vi "Motion-Intialize-Drives.vi"(8 "error in (no error)":errorcluster, 11 "Motion-ControlAll in":refnum<class "Motion-ControlAll.lvclass">) -> (0 "error out":errorcluster, 3 "Motion-ControlAll out":refnum<class "Motion-ControlAll.lvclass">)   [LabVIEW 2013, in "Motion-ControlAll.lvclass"]
uses:
  Motion-ControlAll.lvclass
  Motion-ControlAll.lvclass/Motion-ControlAll.ctl
  <vilib>/addons/_LabVIEW Style Book/Utilities/Style Book Utilities.lvlib
panel:
  out "Normalizing Data":u8(slide) scale=0.0..38.0
  out "STOP":bool
  # "Please wait while Motors Initialize"
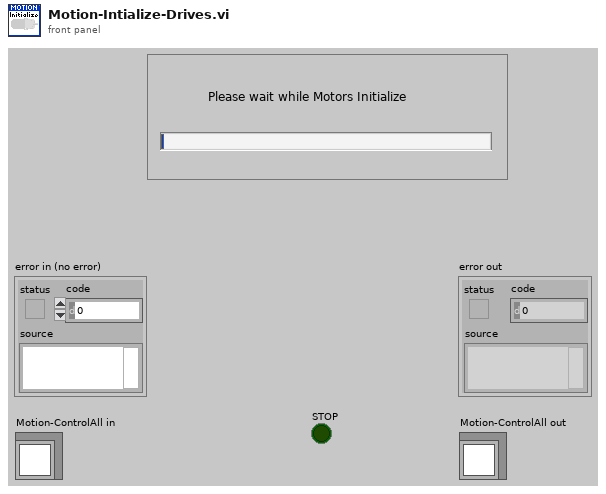
[diagram p1: front panel]
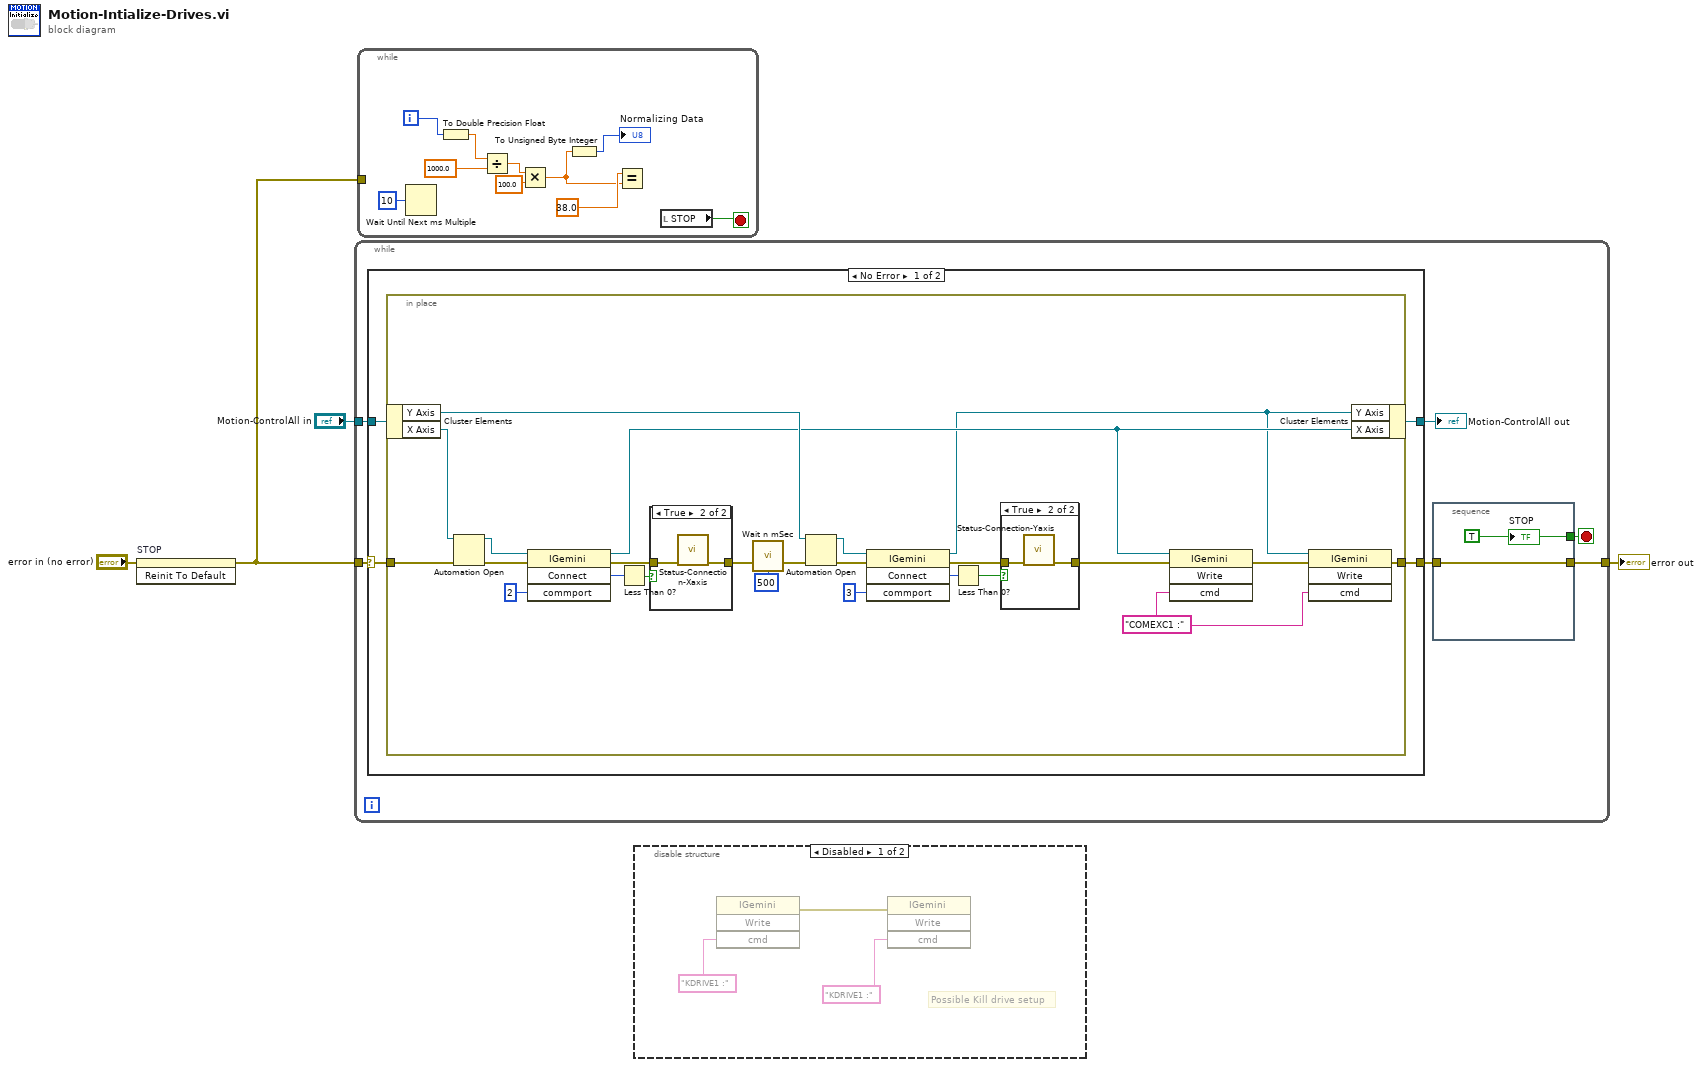
[diagram p0: block diagram]
diagram:
  n1 = invoke on="STOP" class="Bool (strict)" method="Reinit To Default"(error in="error in (no error)") -> (error out=w1:errorcluster)  [unwired: 2 in, 2 out]
  n2 = while {
    tunnel: w1 -> [w9]
    tunnel: [w6] -> w4
    tunnel: "Motion-ControlAll in" -> [w5]
    stop <- w7 stop-if-true
    n3 = case shown="No Error" w9 {
      selector: w9 -> [w15 w48]
      tunnel: [w14 w48] -> w8
      tunnel: [w13 w47] -> w10
      tunnel: w5 -> [w16 w47]
      frame No Error {
        n4 = in-place {
          in-place-border: w15 -> [w40]
          in-place-border: [w31] -> w14
          w33 = "COMEXC1 :" ("cmd")
          n5 = in-place-cluster #1(w16) -> ("Y Axis"=w22:refnum<k7>, "X Axis"=w32:refnum<k7>)
          n6 = Automation Open(error in (no error)=w40, Automation Refnum=w32) -> (Automation Refnum=w37:refnum<k7>, error out=w38:errorcluster)  [unwired: 2 in]
          n7 = invoke class="IGemini" method="Connect"(reference=w37, error in=w38, "commport"=i16 2) -> (reference out=w21:refnum<k7>, error out=w36:errorcluster, "Connect"=w35:i16)  [unwired: 1 in, 1 out]
          n8 = Less Than 0?(x=w35) -> (x < 0?=w30:bool)
          n9 = case shown="True" w30 {
            tunnel: w36 -> [w44 w46]
            tunnel: [w44 w45] -> w19
            frame False {
            }
            frame True {
              n10 = call "Status-Connection-Xaxis.vi"("error in"=w46) -> ("error out"=w45:errorcluster)  [unwired: 10 in]
            }
          }
          n11 = call <vilib>:"Wait n mSec.vi"("error in (no error)"=w19, "Milliseconds to Wait (500)"=u32 500) -> ("error out"=w18:errorcluster)  [unwired: 13 in]
          n12 = Automation Open(error in (no error)=w18, Automation Refnum=w22) -> (Automation Refnum=w26:refnum<k7>, error out=w27:errorcluster)  [unwired: 2 in]
          n13 = invoke class="IGemini" method="Connect"(reference=w26, error in=w27, "commport"=i16 3) -> (reference out=w20:refnum<k7>, error out=w24:errorcluster, "Connect"=w29:i16)  [unwired: 1 in, 1 out]
          n14 = Less Than 0?(x=w29) -> (x < 0?=w25:bool)
          n15 = case shown="True" w25 {
            tunnel: w24 -> [w41 w43]
            tunnel: [w41 w42] -> w23
            frame False {
            }
            frame True {
              n16 = call "Status-Connection-Yaxis.vi"("error in"=w43) -> ("error out"=w42:errorcluster)  [unwired: 10 in]
            }
          }
          n17 = invoke class="IGemini" method="Write"(reference=w21, error in=w23, "cmd"=w33) -> (error out=w34:errorcluster)  [unwired: 1 in, 3 out]
          n18 = invoke class="IGemini" method="Write"(reference=w20, error in=w34, "cmd"=w33) -> (error out=w31:errorcluster)  [unwired: 1 in, 3 out]
          n19 = in-place-cluster #1("Y Axis"=w20, "X Axis"=w21) -> (w13:refnum<class "Motion-ControlAll.lvclass">)
        }
      }
      frame Error {
      }
    }
    "Motion-ControlAll out" <- w10
    n20 = stacked-sequence {
      tunnel: w8 -> [w11]
      tunnel: [w12] -> w7
      tunnel: [w11] -> w6
      frame #0 {
        w12 = TRUE
        "STOP" <- w12
      }
    }
  }
  "error out" <- w4
  n21 = while {
    tunnel: w1 -> [_]
    i -> [w57]
    stop <- w49 stop-if-true
    n22 = Wait Until Next ms Multiple(millisecond multiple=u32 10) -> ()  [unwired: 1 out]
    n23 = To Double Precision Float(number=w57) -> (double precision float=w56:dbl)
    n24 = Divide(x=w56, y=1000.0) -> (x/y=w54:dbl)
    n25 = Multiply(x=w54, y=100.0) -> (x*y=w50:dbl)
    n26 = To Unsigned Byte Integer(number=w50) -> (unsigned 8bit integer=→"Normalizing Data":u8)
    n27 = Equal?(x=38.0, y=w50) -> ()  [unwired: 1 out]
    n28 = local read "STOP"() -> (w49:bool)
  }
  n29 = disable-structure shown="Disabled" {
    frame Disabled {
      # "Possible Kill drive setup"
      n30 = invoke class="IGemini" method="Write"("cmd"="KDRIVE1 :") -> (reference=w63:refnum<k7>, error in=w62:errorcluster, error out=w59:errorcluster)  [unwired: 1 in, 3 out]
      n31 = invoke class="IGemini" method="Write"(error in=w59, "cmd"="KDRIVE1 :") -> ()  [unwired: 2 in, 4 out]
    }
    frame Enabled {
    }
  }
